vi "因子编码配置表.vi"(11 "参数数值":T1={"CODMn"=TRUE, "CODCr"=TRUE, "DO"=TRUE, "铜"=TRUE, "PH"=TRUE, "氨氮"=TRUE, "比电导率"=TRUE, "水温"=TRUE, "COD"=TRUE, "浊度"=TRUE, "总氮"=TRUE, "总磷"=TRUE, "叶绿素a"=TRUE, "藻密度"=TRUE, "水位"=TRUE, "流速"=TRUE, "瞬时流量"=TRUE, "累积流量"=TRUE, "亚硝氮"=TRUE, "硫化物"=TRUE, "ORP"=TRUE, "铅"=TRUE, "镉"=TRUE, "锌"=TRUE, "镍"=TRUE, "锰"=TRUE, "汞"=TRUE, "气温"=TRUE, "气压"=TRUE, "风速"=TRUE, "风向"=TRUE}) -> ()   [LabVIEW 2016]
uses:
  <vilib>/Utility/config.llb/NI_LVConfig.lvlib
panel:
  in  "确定":bool caption="返回"
  in  "返回":bool
  in  "配置表格":string[][](table)
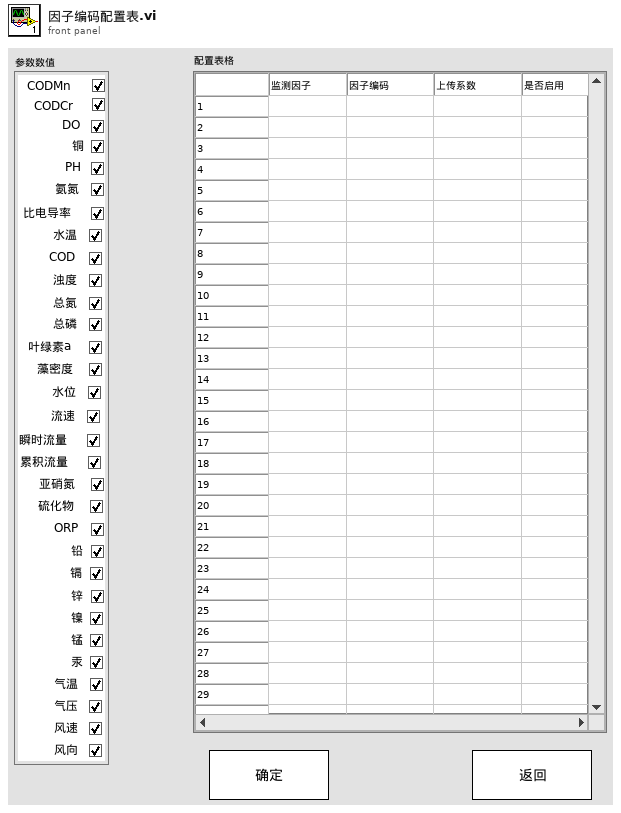
[diagram p1: front panel]
types:
  T1 = cluster{"CODMn":bool, "CODCr":bool, "DO":bool, "铜":bool, "PH":bool, "氨氮":bool, "比电导率":bool, "水温":bool, "COD":bool, "浊度":bool, "总氮":bool, "总磷":bool, "叶绿素a":bool, "藻密度":bool, "水位":bool, "流速":bool, "瞬时流量":bool, "累积流量":bool, "亚硝氮":bool, "硫化物":bool, "ORP":bool, "铅":bool, "镉":bool, "锌":bool, "镍":bool, "锰":bool, "汞":bool, "气温":bool, "气压":bool, "风速":bool, "风向":bool}
  T2 = typedef "NI_LVConfig.lvlib/Config Data RefNum.ctl" = refnum<k1>
  T3 = cluster{"[0]":string, "[1]":string, "[2]":string, "[3]":string, "[4]":string, "[5]":string, "[6]":string, "[7]":string, "[8]":string, "[9]":string, "[10]":string, "[11]":string, "[12]":string, "[13]":string, "[14]":string, "[15]":string, "[16]":string, "[17]":string, "[18]":string, "[19]":string, "[20]":string, "[21]":string, "[22]":string, "[23]":string, "[24]":string, "[25]":string, "[26]":string, "[27]":string, "[28]":string, "[29]":string, "[30]":string}
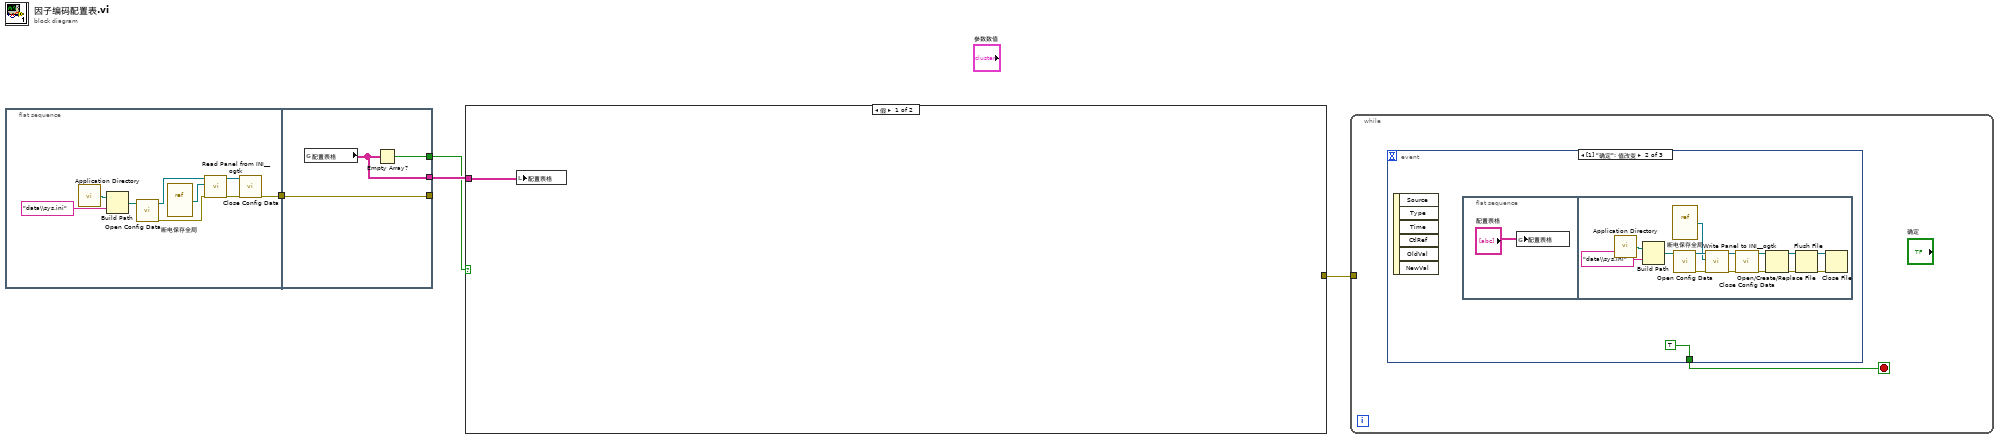
[diagram p0: block diagram]
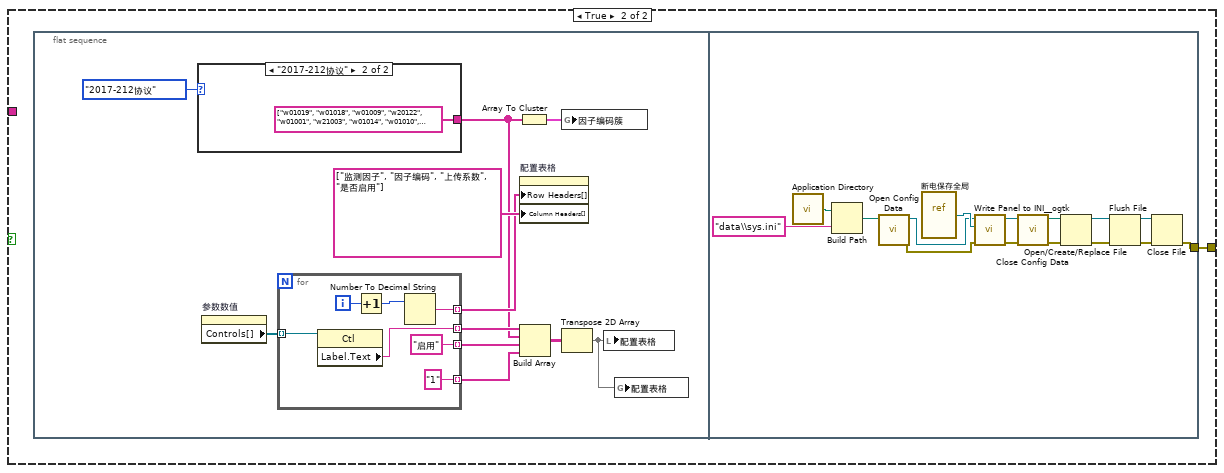
[diagram p2: hidden frame]
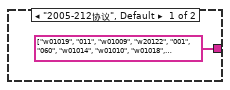
[diagram p3: hidden frame]
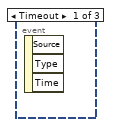
[diagram p4: hidden frame]
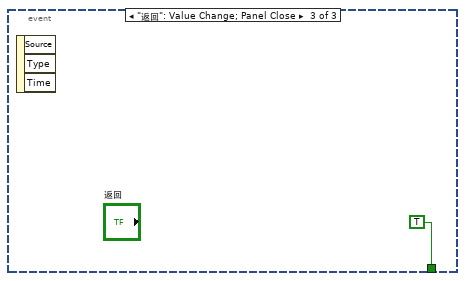
[diagram p5: hidden frame]
diagram:
  n1 = flat-sequence {
    tunnel: [w5] -> w3
    tunnel: [w16] -> _
    tunnel: w3 -> [w16]
    tunnel: [w15] -> w2
    tunnel: [w14] -> w1
    frame #0 {
      n2 = call <vilib>:"Application Directory.vi"() -> ("Application Directory"=w9:path)
      n3 = Build Path(base path=w9, name or relative path="data\\sys.ini" ("名称或相对路径")) -> (appended path=w7:path)
      n4 = call <vilib>:"Open Config Data.vi"("configuration file path"=w7) -> ("error out"=w13:errorcluster, "refnum"=w12:T2)  [unwired: 8 in, 1 out]
      n5 = vi-ref "断电保存全局.vi"() -> (w11:refnum<vi>)
      n6 = call <userlib>:"Read Panel from INI__ogtk.vi"("error in (no error)"=w13, "VI ref"=w11, "refnum"=w12) -> ("error out"=w6:errorcluster, "refnum out"=w10:T2)  [unwired: 7 in]
      n7 = call <vilib>:"Close Config Data.vi"("error in (no error)"=w6, "refnum"=w10) -> ("error out"=w5:errorcluster)  [unwired: 8 in, 1 out]
    }
    frame #1 {
      n8 = global read "断电保存全局.vi" "配置表格"() -> (w15:string[][])
      n9 = Empty Array?(array=w15) -> (empty?=w14:bool)
    }
  }
  n10 = case shown="假" w1 {
    tunnel: w2 -> [w17 _]
    tunnel: [_ w18] -> w4
    frame False {
      n11 = local write "配置表格"(w17) -> ()
    }
    frame True {
      n12 = flat-sequence {
        tunnel: [w39] -> w18
        frame #0 {
          n13 = case shown="\"2017-212协议\"" enum16{"2005-212协议", "2017-212协议"}."2017-212协议" ("数据发送协议") {
            tunnel: [string[] ["w01019", "011", "w01009", "w20122", "001", "060", "w01014", "w01010", "w01018", "w01003", "065", "101", "w01016", "w19011", "e01201", "e01202", "B01", "e01204", "w21006", "w21019", "w01100", "w20120", "w20115", "w20123", "w20121", "w20124", "w20111"] string[] ["w01019", "w01018", "w01009", "w20122", "w01001", "w21003", "w01014", "w01010", "w01018", "w01003", "w21001", "w21011", "w01016", "w19011", "e01201", "e01202", "e01203", "e01204", "w21006", "w21019", "w01100", "w20120", "w20115", "w20123", "w20121", "w20124", "w20111", "a01001", "a01006", "a01007", "a01008"]] -> w21
            frame "2005-212协议", Default {
            }
            frame "2017-212协议" {
            }
          }
          n14 = property on="参数数值" class="Clust (严格)"() -> ("Controls[]"=w28:refnum<vi>[])  [unwired: 2 in, 2 out]
          n15 = for {
            tunnel: w28 -> [w38] mode=indexing
            tunnel: [w35] -> w27 mode=indexing
            tunnel: [w34] -> w25 mode=indexing
            tunnel: ["1"] -> w23 mode=indexing
            tunnel: ["启用"] -> w24 mode=indexing
            i -> [w36]
            n16 = property class="Ctl"(reference=w38) -> ("Label.Text"=w34:string)  [unwired: 1 in, 2 out]
            n17 = Increment(x=w36) -> (x+1=w37:i32)
            n18 = Number To Decimal String(number=w37) -> (decimal integer string=w35:string)  [unwired: 1 in]
          }
          n19 = Array To Cluster(array=w21) -> (cluster=w20:T3)
          n20 = property on="配置表格" class="Tbl (严格)"("Row Headers[]"=w27, "Column Headers[]"=string[] ["监测因子", "因子编码", "上传系数", "是否启用"]) -> ()  [unwired: 2 in, 2 out]
          n21 = Build Array(w25, w21, w24, w23) -> (w26:string[][])
          n22 = global write "断电保存全局.vi" "因子编码簇"(w20) -> ()
          n23 = Transpose 2D Array(2D array=w26) -> (transposed array=w19:string[][])
          n24 = local write "配置表格"(w19) -> ()
          n25 = global write "断电保存全局.vi" "配置表格"(w19) -> ()
        }
        frame #1 {
          n26 = call <vilib>:"Application Directory.vi"() -> ("Application Directory"=w40:path)
          n27 = Build Path(base path=w40, name or relative path="data\\sys.ini" ("名称或相对路径")) -> (appended path=w42:path)
          n28 = call <vilib>:"Open Config Data.vi"("configuration file path"=w42) -> ("error out"=w46:errorcluster, "refnum"=w43:T2)  [unwired: 8 in, 1 out]
          n29 = vi-ref "断电保存全局.vi"() -> (w44:refnum<vi>)
          n30 = call <userlib>:"Write Panel to INI__ogtk.vi"("error in (no error)"=w46, "VI ref"=w44, "refnum"=w43) -> ("error out"=w47:errorcluster, "refnum out"=w45:T2)  [unwired: 7 in]
          n31 = call <vilib>:"Close Config Data.vi"("error in (no error)"=w47, "refnum"=w45) -> ("error out"=w52:errorcluster, "file path"=w53:path)  [unwired: 8 in]
          n32 = Open/Create/Replace File(file path (use dialog)=w53, error in=w52) -> (refnum out=w49:refnum<file>, error out=w48:errorcluster)  [unwired: 4 in, 1 out]
          n33 = Flush File(refnum=w49, error in=w48) -> (refnum out=w50:refnum<file>, error out=w51:errorcluster)
          n34 = Close File(refnum=w50, error in=w51) -> (error out=w39:errorcluster)  [unwired: 1 out]
        }
      }
    }
  }
  n35 = while {
    tunnel: w4 -> [_]
    stop <- w54 stop-if-true
    n36 = event shown="[1] \"确定\": 值改变" {
      selector: _ -> [_ _ _]
      dyn-events: _ -> [_ _ _]
      timeout: _ -> [_ _ _]
      tunnel: [_ TRUE TRUE] -> w54
      event Timeout {
        n37 = event-data() -> ()  [unwired: 1 in, 3 out]
      }
      event "确定": Value Change {
        n38 = event-data() -> ()  [unwired: 1 in, 6 out]
        n39 = flat-sequence {
          frame #0 {
            n40 = global write "断电保存全局.vi" "配置表格"("配置表格") -> ()
          }
          frame #1 {
            n41 = call <vilib>:"Application Directory.vi"() -> ("Application Directory"=w70:path)
            n42 = Build Path(base path=w70, name or relative path="data\\sys.ini" ("名称或相对路径")) -> (appended path=w68:path)
            n43 = vi-ref "断电保存全局.vi"() -> (w66:refnum<vi>)
            n44 = call <vilib>:"Open Config Data.vi"("configuration file path"=w68) -> ("error out"=w64:errorcluster, "refnum"=w67:T2)  [unwired: 8 in, 1 out]
            n45 = call <userlib>:"Write Panel to INI__ogtk.vi"("error in (no error)"=w64, "VI ref"=w66, "refnum"=w67) -> ("error out"=w63:errorcluster, "refnum out"=w65:T2)  [unwired: 7 in]
            n46 = call <vilib>:"Close Config Data.vi"("error in (no error)"=w63, "refnum"=w65) -> ("error out"=w58:errorcluster, "file path"=w57:path)  [unwired: 8 in]
            n47 = Open/Create/Replace File(file path (use dialog)=w57, error in=w58) -> (refnum out=w61:refnum<file>, error out=w62:errorcluster)  [unwired: 4 in, 1 out]
            n48 = Flush File(refnum=w61, error in=w62) -> (refnum out=w60:refnum<file>, error out=w59:errorcluster)
            n49 = Close File(refnum=w60, error in=w59) -> ()  [unwired: 2 out]
          }
        }
      }
      event "返回": Value Change; Panel Close {
        n50 = event-data() -> ()  [unwired: 1 in, 3 out]
      }
    }
  }
